vi "toml_value_datetime.vi"(5 "operation":T1, 6 "modifiers":u16 format="%016b", 7 "section":string[](array[string]), 8 "error in (no error)":errorcluster, 9 "value in":timestamp format="%<%Y-%m-%d %H:%M:%S%6u>T", 10 "key":string[](array[string]), 11 "path in":path) -> (0 "error out":errorcluster, 1 "value out":timestamp format="%<%Y-%m-%d %H:%M:%S%6u>T", 2 "exists?":bool, 3 "path out":path)   [LabVIEW 2017]
uses:
  toml_value_operation.ctl
  toml_fg_action.ctl
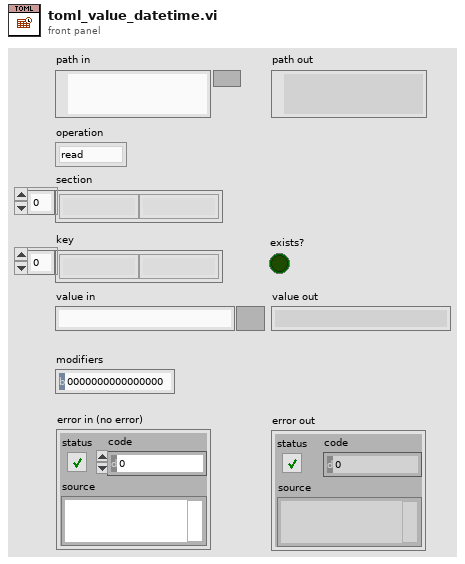
[diagram p1: front panel]
types:
  T1 = typedef "toml_value_operation.ctl" = enum8{"read", "write"}
  T2 = typedef "toml_fg_action.ctl" = enum8{"null", "get", "set", "pop", "import", "export", "drop", "sections", "keys", "remove"}
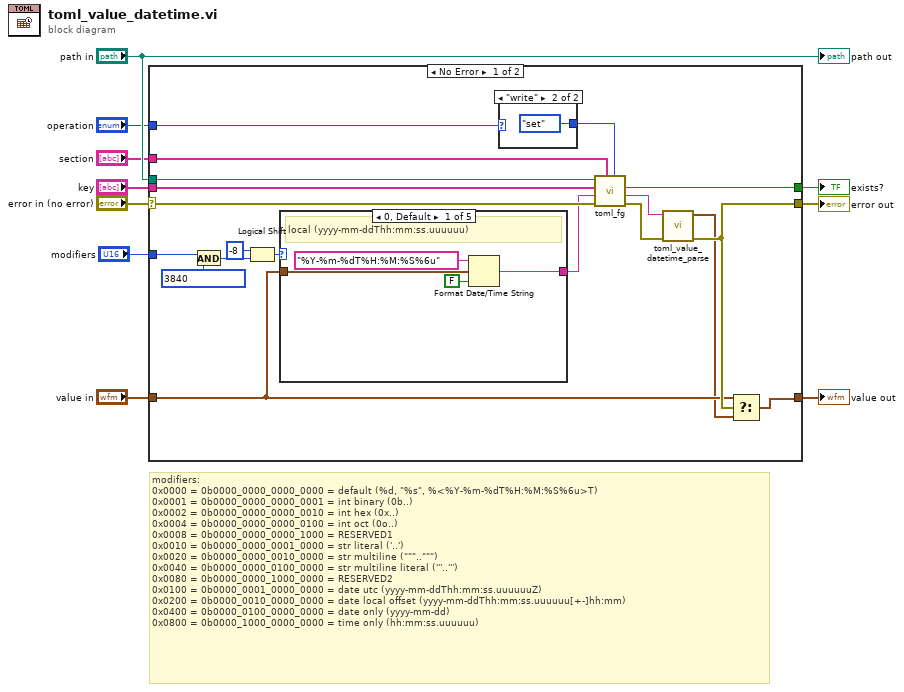
[diagram p0: block diagram]
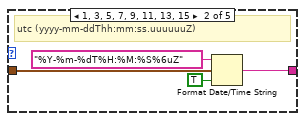
[diagram p2: hidden frame]
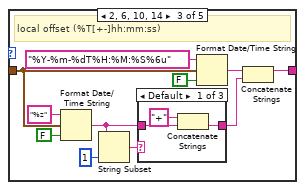
[diagram p3: hidden frame]
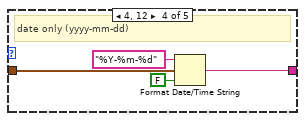
[diagram p6: hidden frame]
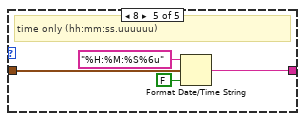
[diagram p7: hidden frame]
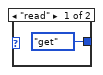
[diagram p8: hidden frame]
diagram:
  # "modifiers:\n0x0000 = 0b0000_0000_0000_0000 = default (%d, \"%s\", %<%Y-%m-%dT%H:%M:%S%6u>T)\n0x0001 = 0b0000_0000_0000_0001 = int binary (0b..)\n0x0002 = 0b0000_0000_0000_0010 = int hex (0x..)\n0x0004 = 0b0000_0000_0000_0100 = int oct (0o..)\n0x0008 = 0b0000_0000_0000_1000 = RESERVED1\n0x0010 = 0b0000_0000_0001_0000 = str literal ('..')\n0x0020 = 0b0000_0000_0010_0000 = str multiline (\"\"\"..\"\"\")\n0x0040 = 0b0000_0000_0100_0000 = str multiline literal ('''..''')\n0x0080 = 0b0000_0000_1000_0000 = RESERVED2\n0x0100 = 0b0000_0001_0000_0000 = date utc (yyyy-mm-ddThh:mm:ss.uuuuuuZ)\n0x0200 = 0b0000_0010_0000_0000 = date local offset (yyyy-mm-ddThh:mm:ss.uuuuuu[+-]hh:mm)\n0x0400 = 0b0000_0100_0000_0000 = date only (yyyy-mm-dd)\n0x0800 = 0b0000_1000_0000_0000 = time only (hh:mm:ss.uuuuuu)"
  n1 = case shown="No Error" "error in (no error)" {
    selector: "error in (no error)" -> [w29 w65]
    tunnel: [w14 w65] -> w9
    tunnel: "path in" -> [w28 _]
    tunnel: "operation" -> [w26 _]
    tunnel: "section" -> [w25 _]
    tunnel: "key" -> [w24 _]
    tunnel: [w23 _] -> w4
    tunnel: [w11 w64] -> w3
    tunnel: "value in" -> [w13 w64]
    tunnel: "modifiers" -> [w22 _]
    frame No Error {
      n2 = And(x=w22, y=u16 3840) -> (x .and. y?=w20:u16)
      n3 = Logical Shift(y=i16 -8, x=w20) -> (x << y=w17:u16)
      n4 = case shown="0, Default" w17 {
        tunnel: w13 -> [w33 w36 w39 w56 w59]
        tunnel: [w32 w35 w40 w55 w58] -> w18
        frame 0, Default {
          # "local (yyyy-mm-ddThh:mm:ss.uuuuuu)"
          n5 = Format Date/Time String(time format string (%c)="%Y-%m-%dT%H:%M:%S%6u", seconds (now)=w33, UTC format=FALSE) -> (date/time string=w32:string)
        }
        frame 1, 3, 5, 7, 9, 11, 13, 15 {
          # "utc (yyyy-mm-ddThh:mm:ss.uuuuuuZ)"
          n6 = Format Date/Time String(time format string (%c)="%Y-%m-%dT%H:%M:%S%6uZ", seconds (now)=w36, UTC format=TRUE) -> (date/time string=w35:string)
        }
        frame 2, 6, 10, 14 {
          # "local offset (%T[+-]hh:mm:ss)"
          n7 = Format Date/Time String(time format string (%c)="%z", seconds (now)=w39, UTC format=FALSE) -> (date/time string=w43:string)
          n8 = String Subset(string=w43, length (rest)=1 ("length (rest)")) -> (substring=w44:string)  [unwired: 1 in]
          n9 = case shown="Default" w44 {
            tunnel: w43 -> [w51 w52 w53]
            tunnel: [w50 w52 w53] -> w42
            frame Default {
              n10 = Concatenate Strings("+" ("string"), w51) -> (w50:string)
            }
            frame "+" {
            }
            frame "-" {
            }
          }
          n11 = Format Date/Time String(time format string (%c)="%Y-%m-%dT%H:%M:%S%6u", seconds (now)=w39, UTC format=FALSE) -> (date/time string=w48:string)
          n12 = Concatenate Strings(w48, w42) -> (w40:string)
        }
        frame 4, 12 {
          # "date only (yyyy-mm-dd)"
          n13 = Format Date/Time String(time format string (%c)="%Y-%m-%d", seconds (now)=w56, UTC format=FALSE) -> (date/time string=w55:string)
        }
        frame 8 {
          # "time only (hh:mm:ss.uuuuuu)"
          n14 = Format Date/Time String(time format string (%c)="%H:%M:%S%6u", seconds (now)=w59, UTC format=FALSE) -> (date/time string=w58:string)
        }
      }
      n15 = case shown="\"write\"" w26 {
        tunnel: [toml_fg_action."get" ("action") toml_fg_action."set" ("action")] -> w27
        frame "read" {
        }
        frame "write" {
        }
      }
      n16 = call "toml_fg.vi"("action"=w27, "section"=w25, "error in (no error)"=w29, "value in"=w18, "key"=w24, "path in"=w28) -> ("error out"=w16:errorcluster, "value out"=w15:string, "exists?"=w23:bool)  [unwired: 2 in, 1 out]
      n17 = call "toml_value_datetime_parse.vi"("error in (no error)"=w16, "value"=w15) -> ("error out"=w14:errorcluster, "time stamp"=w12:timestamp)  [unwired: 8 in]
      n18 = Select(t=w13, s=w14, f=w12) -> (s? t:f=w11:timestamp)
    }
    frame Error {
    }
  }
  "error out" <- w9
  "value out" <- w3
  "exists?" <- w4
  "path out" <- "path in"
